vi "ChordsRecognition.vi"() -> ()   [LabVIEW 2021]
uses:
  <vilib>/Utility/NIReport.llb/Report Type.ctl
  <vilib>/numeric/Random Number (Range) I64.vi
  <vilib>/Analysis/baseanly.llb/Real A x B.vi
  <vilib>/numeric/sub_Random U32.vi
  <vilib>/Utility/file.llb/Read Delimited Spreadsheet (DBL).vi
  <vilib>/addons/_office/excel.llb/Excel Easy Table (str).vi
  <vilib>/Analysis/Matrix/Numeric/Conversions/Matrix To Array - RM.vi
  <vilib>/Utility/NIReport.llb/NI_report.lvclass
  <vilib>/Analysis/NI_AALBase.lvlib
  <vilib>/Analysis/Matrix/NI_Matrix.lvlib
  <vilib>/Utility/NIReport.llb/NI_ReportGenerationCore.lvlib
  <vilib>/Utility/NIReport.llb/Excel/NI_Excel.lvclass
  <vilib>/addons/_office/NI_ReportGenerationToolkit.lvlib
panel:
  out "n":i32
  in  "Save":bool
  in  "Array":bool[](array[boolean])
  in  "Saved":bool
  in  "index":i32
  out "Y_ideal":dbl[][][](array[numeric])
  out "Playing":string
  out "Keys":bool[][](array[boolean])
  out "la#":bool
  out "sol#":bool
  out "fa#":bool
  out "re#":bool
  out "do#":bool
  out "si":bool
  out "la":bool
  out "sol":bool
  out "fa":bool
  out "mi":bool
  out "re":bool
  out "do":bool
  out "Confidence":dbl
  out "min value":dbl
  out "max value":dbl
  in  "Random":bool
  in  "Output":i32=1
  in  "2th layer":i32=2
  in  "1th layer":i32=3
  in  "Predict":bool
  out "Error":dbl[](array[numeric])
  in  "W1":dbl[][](array[numeric])
  out "Y":dbl[][][](array[numeric])
  in  "Learn?":bool
  in  "Lr":dbl
  in  "stop":bool
  in  "Bias 2":dbl[][](array[numeric]) format="%#_13g"
  in  "Bias 3":dbl[][](array[numeric]) format="%#_13g"
  in  "Bias 1":dbl[][](array[numeric]) format="%#_13g"
  in  "W2":dbl[][](array[numeric])
  in  "W3":dbl[][](array[numeric])
  out "C":i16[][](array[numeric])
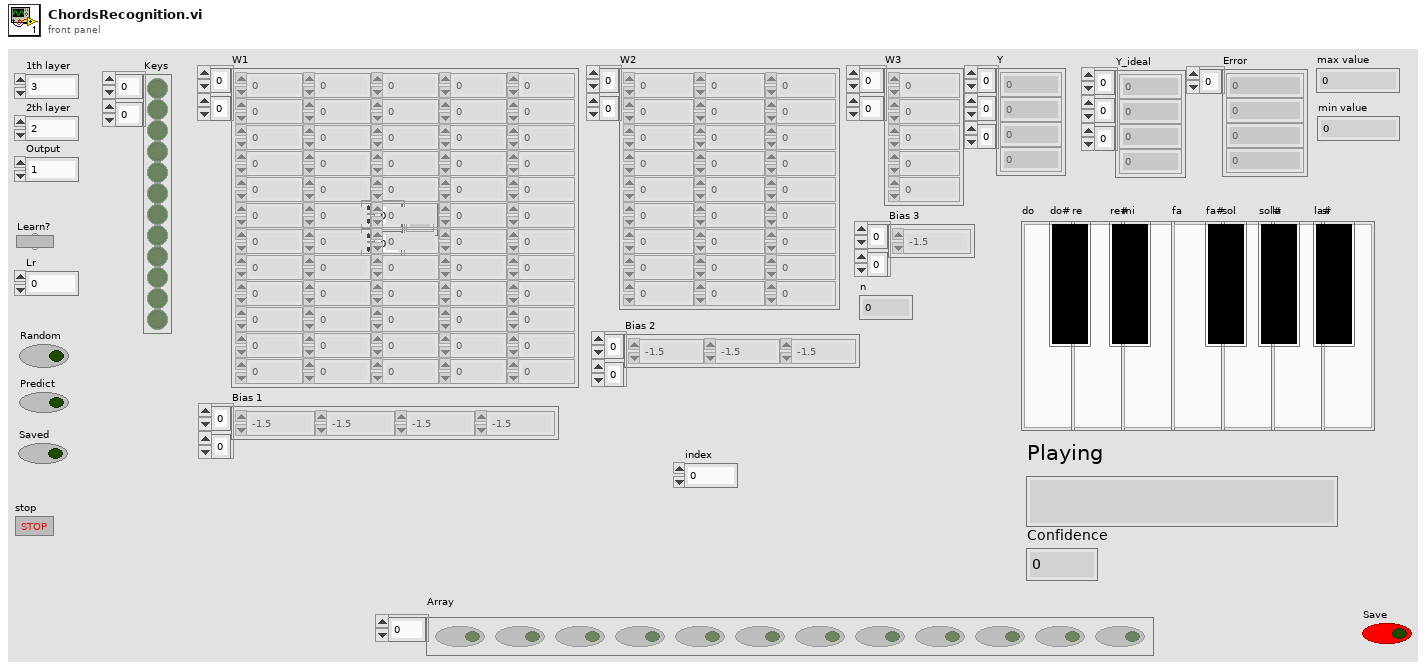
[diagram p1: front panel]
types:
  T1 = typedef "NI_ReportGenerationCore.lvlib/Report Type.ctl" = enum16{"HTML", "Word", "Excel"}
  T2 = typedef "NI_Matrix.lvlib/RealMatrix.ctl" = dbl[][]
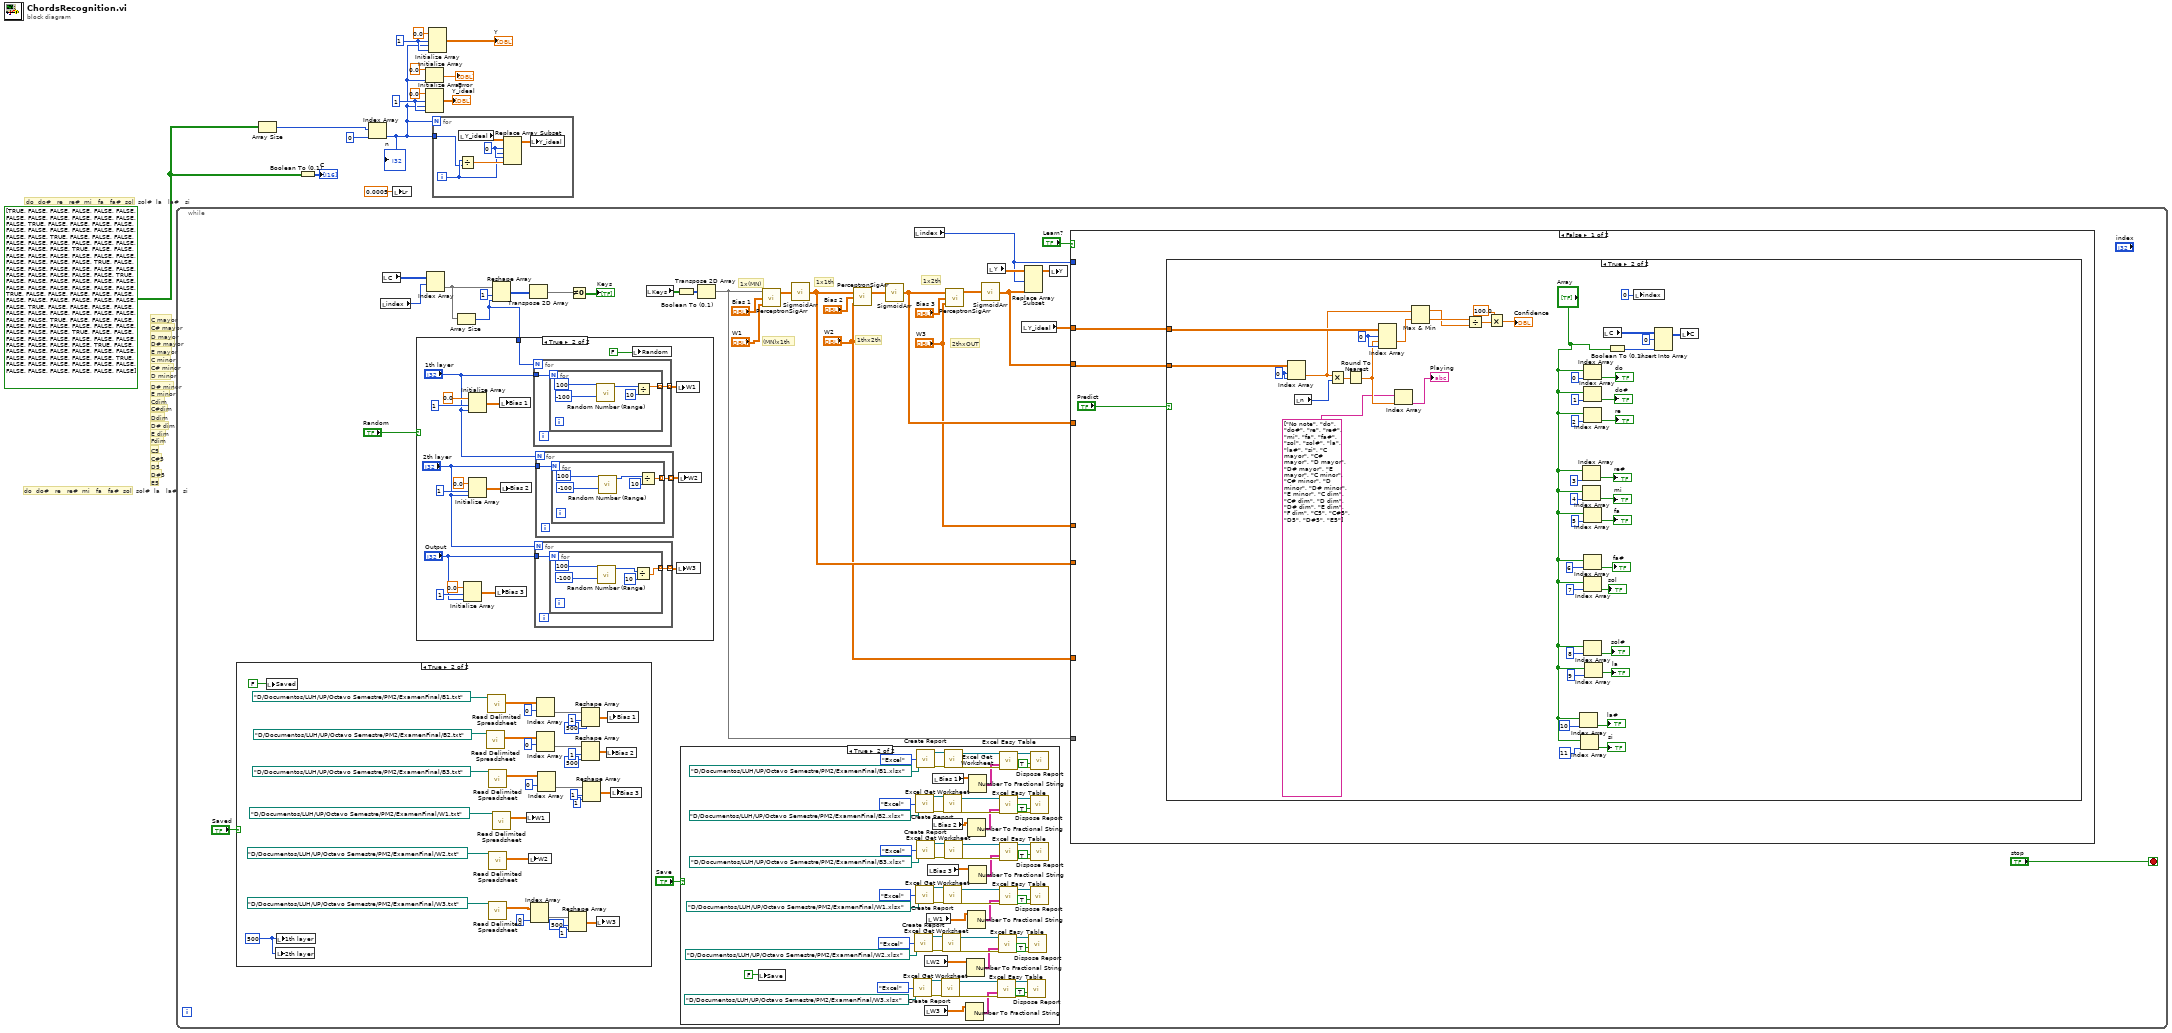
[diagram p0: block diagram]
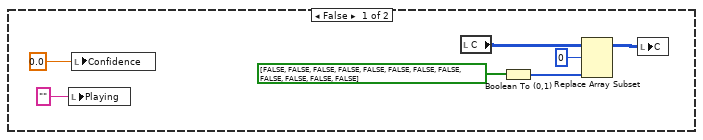
[diagram p5: hidden frame]
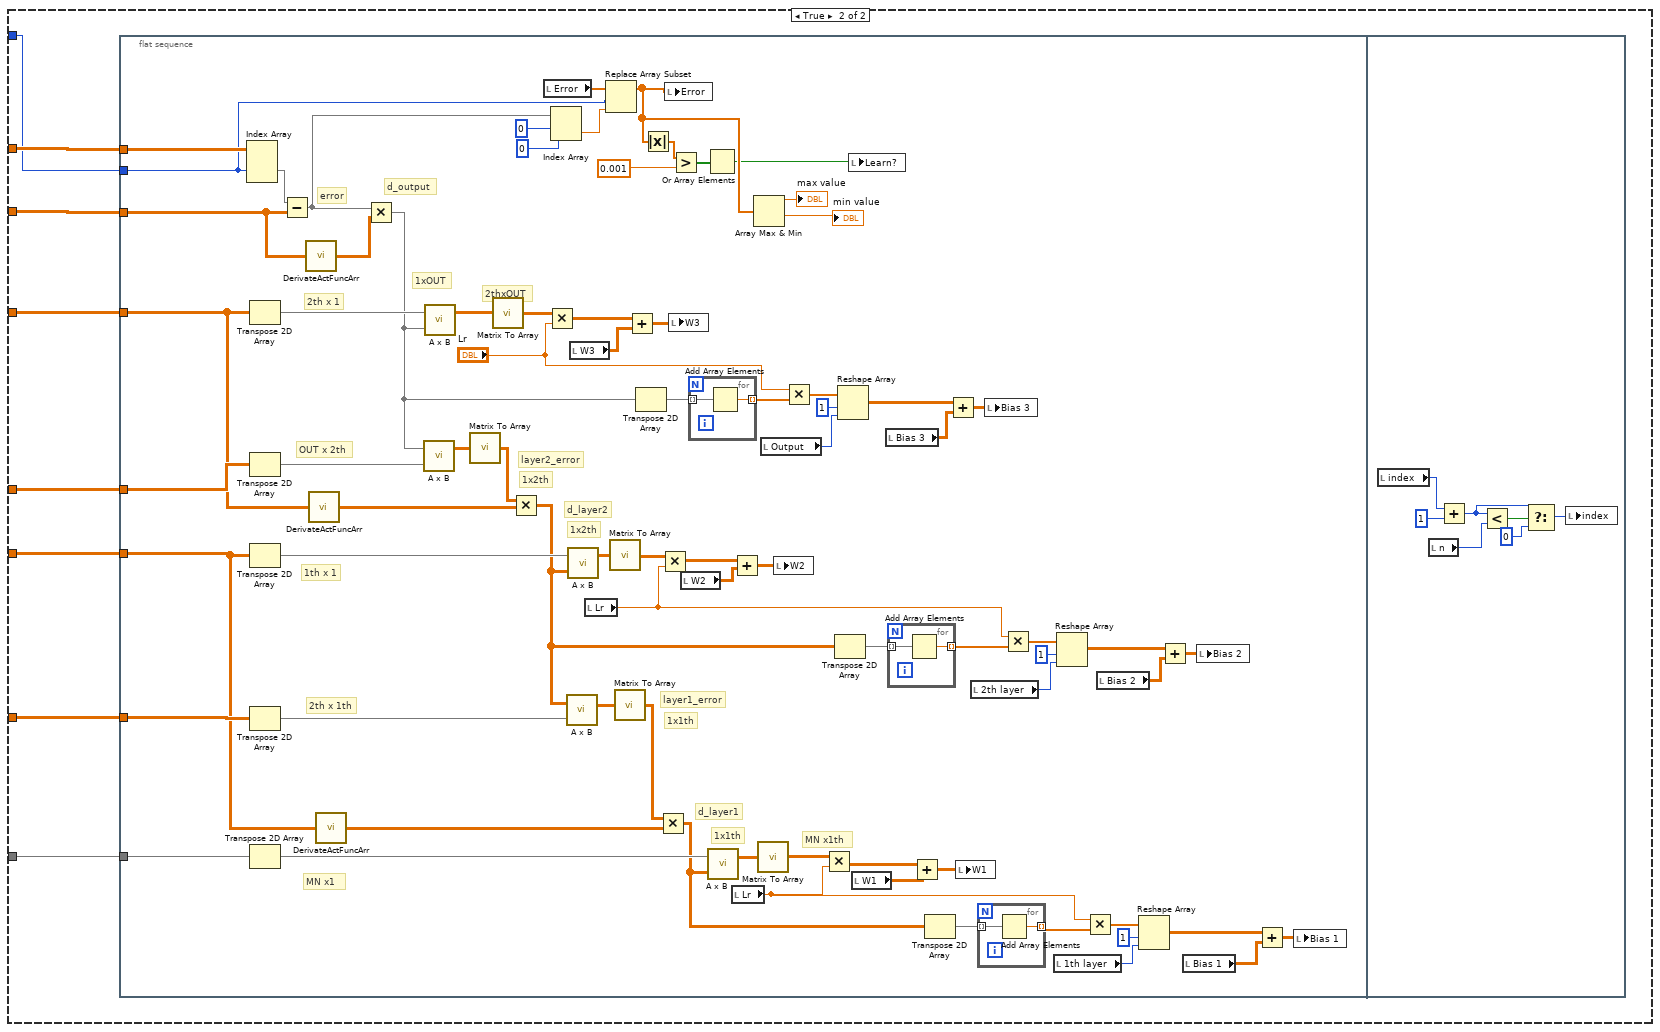
[diagram p6: hidden frame]
diagram:
  w1 = bool[][] [[TRUE, FALSE, FALSE, FALSE, FALSE, FALSE, FALSE, FALSE, FALSE, FALSE, FALSE, FALSE], [FALSE, TRUE, FALSE, FALSE, FALSE, FALSE, FALSE, FALSE, FALSE, FALSE, FALSE, FALSE], [FALSE, FALSE, TRUE, FALSE, FALSE, FALSE, FALSE, FALSE, FALSE, FALSE, FALSE, FALSE], [FALSE, FALSE, FALSE, TRUE, FALSE, FALSE, FALSE, FALSE, FALSE, FALSE, FALSE, FALSE], [FALSE, FALSE, FALSE, FALSE, TRUE, FALSE, FALSE, FALSE, FALSE, FALSE, FALSE, FALSE], [FALSE, FALSE, FALSE, FALSE, FALSE, TRUE, FALSE, FALSE, FALSE, FALSE, FALSE, FALSE], [FALSE, FALSE, FALSE, FALSE, FALSE, FALSE, TRUE, FALSE, FALSE, FALSE, FALSE, FALSE], [FALSE, FALSE, FALSE, FALSE, FALSE, FALSE, FALSE, TRUE, FALSE, FALSE, FALSE, FALSE], [FALSE, FALSE, FALSE, FALSE, FALSE, FALSE, FALSE, FALSE, TRUE, FALSE, FALSE, FALSE], [FALSE, FALSE, FALSE, FALSE, FALSE, FALSE, FALSE, FALSE, FALSE, TRUE, FALSE, FALSE], [FALSE, FALSE, FALSE, FALSE, FALSE, FALSE, FALSE, FALSE, FALSE, FALSE, TRUE, FALSE], [FALSE, FALSE, FALSE, FALSE, FALSE, FALSE, FALSE, FALSE, FALSE, FALSE, FALSE, TRUE], [FALSE, FALSE, FALSE, FALSE, FALSE, FALSE, FALSE, FALSE, FALSE, FALSE, FALSE, FALSE]]
  w7 = 1 ("dimension size")
  w13 = 1 ("dimension size")
  # "do  do#   re   re#  mi   fa   fa#  sol  sol#  la   la#   si"
  # "do  do#   re   re#  mi   fa   fa#  sol  sol#  la   la#   si"
  # "D# dim"
  # "D5"
  # "Ddim"
  # "C#5"
  # "C#dim"
  # "C5"
  # "Cdim"
  # "Fdim"
  # "E5"
  # "E dim"
  # "E minor"
  # "E mayor"
  # "D#5"
  # "D# minor"
  # "D# mayor"
  # "D minor"
  # "D mayor"
  # "C# minor"
  # "C# mayor"
  # "C minor"
  # "C mayor"
  n1 = while {
    stop <- "stop" stop-if-true
    # "2thxOUT"
    # "1x2th"
    # "1thx2th"
    # "1x1th"
    # "1x(MN)"
    # "(MN)x1th"
    n2 = case shown="True" "Saved" {
      frame False {
      }
      frame True {
        w140 = 500 ("1th layer")
        n3 = local write "Saved"(FALSE ("Boolean")) -> ()
        n4 = local write "2th layer"(w140) -> ()
        n5 = local write "1th layer"(w140) -> ()
        n6 = call-poly <vilib>:"Read Delimited Spreadsheet.vi"("file path (dialog if empty)"=path "D:/Documentos/LUH/UP/Octavo Semestre/PM2/ExamenFinal/B2.txt" ("template (empty)")) -> ("all rows"=w128:dbl[][])  [unwired: 9 in, 5 out]
        n7 = call-poly <vilib>:"Read Delimited Spreadsheet.vi"("file path (dialog if empty)"=path "D:/Documentos/LUH/UP/Octavo Semestre/PM2/ExamenFinal/B1.txt" ("template (empty)")) -> ("all rows"=w137:dbl[][])  [unwired: 9 in, 5 out]
        n8 = call-poly <vilib>:"Read Delimited Spreadsheet.vi"("file path (dialog if empty)"=path "D:/Documentos/LUH/UP/Octavo Semestre/PM2/ExamenFinal/B3.txt" ("template (empty)")) -> ("all rows"=w121:dbl[][])  [unwired: 9 in, 5 out]
        n9 = call-poly <vilib>:"Read Delimited Spreadsheet.vi"("file path (dialog if empty)"=path "D:/Documentos/LUH/UP/Octavo Semestre/PM2/ExamenFinal/W3.txt" ("template (empty)")) -> ("all rows"=w119:dbl[][])  [unwired: 9 in, 5 out]
        n10 = call-poly <vilib>:"Read Delimited Spreadsheet.vi"("file path (dialog if empty)"=path "D:/Documentos/LUH/UP/Octavo Semestre/PM2/ExamenFinal/W2.txt" ("template (empty)")) -> ("all rows"=w138:dbl[][])  [unwired: 9 in, 5 out]
        n11 = call-poly <vilib>:"Read Delimited Spreadsheet.vi"("file path (dialog if empty)"=path "D:/Documentos/LUH/UP/Octavo Semestre/PM2/ExamenFinal/W1.txt" ("template (empty)")) -> ("all rows"=w139:dbl[][])  [unwired: 9 in, 5 out]
        n12 = local write "W1"(w139) -> ()
        n13 = local write "W2"(w138) -> ()
        n14 = Index Array(array=w119, index (col)=0 ("index (row)")) -> (element=w116:dbl[])  [unwired: 1 in]
        n15 = Index Array(array=w137, index (row)=0) -> (element=w135:dbl[])  [unwired: 1 in]
        n16 = Index Array(array=w128, index (row)=0) -> (element=w130:dbl[])  [unwired: 1 in]
        n17 = Index Array(array=w121, index (row)=0) -> (element=w124:dbl[])  [unwired: 1 in]
        n18 = Reshape Array(w116, 500 ("dimension size"), 1 ("dimension size")) -> (w115:dbl[][])
        n19 = Reshape Array(w135, 1 ("dimension size"), 500 ("dimension size")) -> (w132:dbl[][])
        n20 = Reshape Array(w130, 1 ("dimension size"), 500 ("dimension size")) -> (w127:dbl[][])
        n21 = Reshape Array(w124, 1 ("dimension size"), 1 ("dimension size")) -> (w120:dbl[][])
        n22 = local write "W3"(w115) -> ()
        n23 = local write "Bias 2"(w127) -> ()
        n24 = local write "Bias 1"(w132) -> ()
        n25 = local write "Bias 3"(w120) -> ()
      }
    }
    n26 = local read "index"() -> (w17:i32)
    n27 = local read "C"() -> (w21:i16[][])
    n28 = Index Array(array=w21, index (row)=w17) -> (element=w16:i16[])  [unwired: 1 in]
    n29 = Array Size(array=w16) -> (size(s)=w15:i32)
    n30 = case shown="True" "Random" {
      tunnel: w15 -> [_ w163]
      frame False {
      }
      frame True {
        n31 = Initialize Array(0.0 ("element"), 1 ("dimension size"), "Output") -> (w148:dbl[][])
        n32 = Initialize Array(0.0 ("element"), 1 ("dimension size"), "1th layer") -> (w162:dbl[][])
        n33 = Initialize Array(0.0 ("element"), 1 ("dimension size"), "2th layer") -> (w157:dbl[][])
        n34 = local write "Bias 3"(w148) -> ()
        n35 = local write "Bias 1"(w162) -> ()
        n36 = local write "Bias 2"(w157) -> ()
        n37 = for {
          N: w163 -> [_]
          tunnel: "1th layer" -> [w180]
          tunnel: [w179] -> w159 mode=indexing
          n38 = for {
            N: w180 -> [_]
            tunnel: [w182] -> w179 mode=indexing
            n39 = call-poly <vilib>:"Random Number (Range).vi"("lower bound (-100)"=i64 -100, "upper bound (100)"=i64 100) -> ("number"=w183:i64)  [unwired: 9 in]
            n40 = Divide(x=w183, y=i64 10) -> (x/y=w182:dbl)
          }
        }
        n41 = for {
          N: "2th layer" -> [_]
          tunnel: "Output" -> [w166]
          tunnel: [w165] -> w152 mode=indexing
          n42 = for {
            N: w166 -> [_]
            tunnel: [w167] -> w165 mode=indexing
            n43 = call-poly <vilib>:"Random Number (Range).vi"("lower bound (-100)"=i64 -100, "upper bound (100)"=i64 100) -> ("number"=w168:i64)  [unwired: 9 in]
            n44 = Divide(x=w168, y=i64 10) -> (x/y=w167:dbl)
          }
        }
        n45 = for {
          N: "1th layer" -> [_]
          tunnel: "2th layer" -> [w173]
          tunnel: [w172] -> w153 mode=indexing
          n46 = for {
            N: w173 -> [_]
            tunnel: [w175] -> w172 mode=indexing
            n47 = call-poly <vilib>:"Random Number (Range).vi"("lower bound (-100)"=i64 -100, "upper bound (100)"=i64 100) -> ("number"=w174:i64)  [unwired: 9 in]
            n48 = Divide(x=w174, y=i64 10) -> (x/y=w175:dbl)
          }
        }
        n49 = local write "Random"(FALSE ("Init")) -> ()
        n50 = local write "W1"(w159) -> ()
        n51 = local write "W3"(w152) -> ()
        n52 = local write "W2"(w153) -> ()
      }
    }
    n53 = Reshape Array(w16, 1 ("dimension size"), w15) -> (w19:i16[][])
    n54 = Transpose 2D Array(2D array=w19) -> (transposed array=w18:i16[][])
    n55 = Not Equal To 0?(x=w18) -> (x != 0?=→"Keys":bool[][])
    n56 = local read "Keys"() -> (w29:bool[][])
    n57 = Boolean To (0,1)(Boolean=w29) -> (0, 1=w30:i16[][])
    n58 = case shown="True" "Save" {
      frame False {
      }
      frame True {
        n59 = local write "Save"(FALSE ("Save")) -> ()
        n60 = call <vilib>:"Create Report.vi"("report type"=Report_Type."Excel", "template (empty)"=path "D:/Documentos/LUH/UP/Octavo Semestre/PM2/ExamenFinal/W3.xlsx") -> ("report out"=w61:refnum<class "NI_report.lvclass">, "error out"=w60:errorcluster)  [unwired: 12 in]
        n61 = call <vilib>:"Create Report.vi"("report type"=Report_Type."Excel", "template (empty)"=path "D:/Documentos/LUH/UP/Octavo Semestre/PM2/ExamenFinal/W2.xlsx") -> ("report out"=w71:refnum<class "NI_report.lvclass">, "error out"=w70:errorcluster)  [unwired: 12 in]
        n62 = call <vilib>:"Create Report.vi"("report type"=Report_Type."Excel", "template (empty)"=path "D:/Documentos/LUH/UP/Octavo Semestre/PM2/ExamenFinal/B2.xlsx") -> ("report out"=w101:refnum<class "NI_report.lvclass">, "error out"=w100:errorcluster)  [unwired: 12 in]
        n63 = call <vilib>:"Create Report.vi"("report type"=Report_Type."Excel", "template (empty)"=path "D:/Documentos/LUH/UP/Octavo Semestre/PM2/ExamenFinal/W1.xlsx") -> ("report out"=w81:refnum<class "NI_report.lvclass">, "error out"=w80:errorcluster)  [unwired: 12 in]
        n64 = call <vilib>:"Create Report.vi"("report type"=Report_Type."Excel", "template (empty)"=path "D:/Documentos/LUH/UP/Octavo Semestre/PM2/ExamenFinal/B1.xlsx") -> ("report out"=w111:refnum<class "NI_report.lvclass">, "error out"=w110:errorcluster)  [unwired: 12 in]
        n65 = call <vilib>:"Create Report.vi"("report type"=Report_Type."Excel", "template (empty)"=path "D:/Documentos/LUH/UP/Octavo Semestre/PM2/ExamenFinal/B3.xlsx") -> ("report out"=w91:refnum<class "NI_report.lvclass">, "error out"=w90:errorcluster)  [unwired: 12 in]
        n66 = local read "W2"() -> (w49:dbl[][])
        n67 = local read "W3"() -> (w48:dbl[][])
        n68 = local read "W1"() -> (w50:dbl[][])
        n69 = local read "Bias 3"() -> (w51:dbl[][])
        n70 = local read "Bias 2"() -> (w52:dbl[][])
        n71 = local read "Bias 1"() -> (w53:dbl[][])
        n72 = call <vilib>:"Excel Get Worksheet.vi"("report in"=w61, "error in (no error)"=w60) -> ("report out"=w59:refnum<class "NI_report.lvclass">, "error out"=w58:errorcluster)  [unwired: 12 in]
        n73 = call <vilib>:"Excel Get Worksheet.vi"("report in"=w71, "error in (no error)"=w70) -> ("report out"=w69:refnum<class "NI_report.lvclass">, "error out"=w68:errorcluster)  [unwired: 12 in]
        n74 = call <vilib>:"Excel Get Worksheet.vi"("report in"=w101, "error in (no error)"=w100) -> ("report out"=w99:refnum<class "NI_report.lvclass">, "error out"=w98:errorcluster)  [unwired: 12 in]
        n75 = call <vilib>:"Excel Get Worksheet.vi"("report in"=w81, "error in (no error)"=w80) -> ("report out"=w79:refnum<class "NI_report.lvclass">, "error out"=w78:errorcluster)  [unwired: 12 in]
        n76 = call <vilib>:"Excel Get Worksheet.vi"("report in"=w111, "error in (no error)"=w110) -> ("report out"=w109:refnum<class "NI_report.lvclass">, "error out"=w108:errorcluster)  [unwired: 12 in]
        n77 = call <vilib>:"Excel Get Worksheet.vi"("report in"=w91, "error in (no error)"=w90) -> ("report out"=w89:refnum<class "NI_report.lvclass">, "error out"=w88:errorcluster)  [unwired: 12 in]
        n78 = Number To Fractional String(number=w48) -> (F-format string=w57:string[][])  [unwired: 3 in]
        n79 = Number To Fractional String(number=w49) -> (F-format string=w67:string[][])  [unwired: 3 in]
        n80 = Number To Fractional String(number=w52) -> (F-format string=w97:string[][])  [unwired: 3 in]
        n81 = Number To Fractional String(number=w50) -> (F-format string=w77:string[][])  [unwired: 3 in]
        n82 = Number To Fractional String(number=w53) -> (F-format string=w107:string[][])  [unwired: 3 in]
        n83 = Number To Fractional String(number=w51) -> (F-format string=w87:string[][])  [unwired: 3 in]
        n84 = call-poly <vilib>:"Excel Easy Table.vi"("report in"=w59, "text data"=w57, "error in (no error)"=w58) -> ("report out"=w56:refnum<class "NI_report.lvclass">, "error out"=w55:errorcluster)  [unwired: 8 in, 3 out]
        n85 = call-poly <vilib>:"Excel Easy Table.vi"("report in"=w69, "text data"=w67, "error in (no error)"=w68) -> ("report out"=w66:refnum<class "NI_report.lvclass">, "error out"=w65:errorcluster)  [unwired: 8 in, 3 out]
        n86 = call-poly <vilib>:"Excel Easy Table.vi"("report in"=w99, "text data"=w97, "error in (no error)"=w98) -> ("report out"=w96:refnum<class "NI_report.lvclass">, "error out"=w95:errorcluster)  [unwired: 8 in, 3 out]
        n87 = call-poly <vilib>:"Excel Easy Table.vi"("report in"=w79, "text data"=w77, "error in (no error)"=w78) -> ("report out"=w76:refnum<class "NI_report.lvclass">, "error out"=w75:errorcluster)  [unwired: 8 in, 3 out]
        n88 = call-poly <vilib>:"Excel Easy Table.vi"("report in"=w109, "text data"=w107, "error in (no error)"=w108) -> ("report out"=w106:refnum<class "NI_report.lvclass">, "error out"=w105:errorcluster)  [unwired: 8 in, 3 out]
        n89 = call-poly <vilib>:"Excel Easy Table.vi"("report in"=w89, "text data"=w87, "error in (no error)"=w88) -> ("report out"=w86:refnum<class "NI_report.lvclass">, "error out"=w85:errorcluster)  [unwired: 8 in, 3 out]
        n90 = call-dynamic "Dispose Report.vi"("report in"=w56, "save changes? (F)"=TRUE, "error in (no error)"=w55) -> ()  [unwired: 12 in, 1 out]
        n91 = call-dynamic "Dispose Report.vi"("report in"=w66, "save changes? (F)"=TRUE, "error in (no error)"=w65) -> ()  [unwired: 12 in, 1 out]
        n92 = call-dynamic "Dispose Report.vi"("report in"=w96, "save changes? (F)"=TRUE, "error in (no error)"=w95) -> ()  [unwired: 12 in, 1 out]
        n93 = call-dynamic "Dispose Report.vi"("report in"=w76, "save changes? (F)"=TRUE, "error in (no error)"=w75) -> ()  [unwired: 12 in, 1 out]
        n94 = call-dynamic "Dispose Report.vi"("report in"=w106, "save changes? (F)"=TRUE, "error in (no error)"=w105) -> ()  [unwired: 12 in, 1 out]
        n95 = call-dynamic "Dispose Report.vi"("report in"=w86, "save changes? (F)"=TRUE, "error in (no error)"=w85) -> ()  [unwired: 12 in, 1 out]
      }
    }
    n96 = Transpose 2D Array(2D array=w30) -> (transposed array=w28:i16[][])
    n97 = call "PerceptronSigArr.vi"("Wa"="W1", "Bias"="Bias 1", "Xa"=w28) -> ("Y"=w41:dbl[][])
    n98 = call "SigmoidArr.vi"("x"=w41) -> ("Sigmoid"=w38:dbl[][])
    n99 = call "PerceptronSigArr.vi"("Wa"="W2", "Bias"="Bias 2", "Xa"=w38) -> ("Y"=w44:dbl[][])
    n100 = call "SigmoidArr.vi"("x"=w44) -> ("Sigmoid"=w36:dbl[][])
    n101 = local read "index"() -> (w26:i32)
    n102 = call "PerceptronSigArr.vi"("Wa"="W3", "Bias"="Bias 3", "Xa"=w36) -> ("Y"=w42:dbl[][])
    n103 = call "SigmoidArr.vi"("x"=w42) -> ("Sigmoid"=w25:dbl[][])
    n104 = local read "Y"() -> (w27:dbl[][][])
    n105 = local read "Y_ideal"() -> (w23:dbl[][][])
    n106 = Replace Array Subset(array=w27, new element=w25, index (dim 1)=w26) -> (w24:dbl[][][])  [unwired: 2 in]
    n107 = local write "Y"(w24) -> ()
    n108 = case shown="False" "Learn?" {
      tunnel: w25 -> [w187 w248]
      tunnel: w23 -> [w186 w249]
      tunnel: w36 -> [_ w246]
      tunnel: "W3" -> [_ w247]
      tunnel: w38 -> [_ w244]
      tunnel: "W2" -> [_ w245]
      tunnel: w28 -> [_ w243]
      tunnel: w26 -> [_ w242]
      frame False {
        n109 = case shown="True" "Predict" {
          tunnel: w187 -> [_ w240]
          tunnel: w186 -> [_ w239]
          frame False {
            n110 = local write "Playing"("" ("Playing")) -> ()
            n111 = local write "Confidence"(0.0 ("Pattern")) -> ()
            n112 = local read "C"() -> (w191:i16[][])
            n113 = Boolean To (0,1)(Boolean=bool[] [FALSE, FALSE, FALSE, FALSE, FALSE, FALSE, FALSE, FALSE, FALSE, FALSE, FALSE, FALSE]) -> (0, 1=w193:i16[])
            n114 = Replace Array Subset(array=w191, new element=w193, index (row)=0) -> (w189:i16[][])  [unwired: 1 in]
            n115 = local write "C"(w189) -> ()
          }
          frame True {
            w238 = 0 ("disabled index (page)")
            w241 = 0 ("index (row)")
            n116 = Index Array(array=w240, index (row)=w241, index (col)=w241) -> (element=w230:dbl)
            n117 = local read "n"() -> (w196:i32)
            n118 = Multiply(x=w230, y=w196) -> (x*y=w234:dbl)
            n119 = Round To Nearest(number=w234) -> (nearest integer value=w229:dbl)
            n120 = Index Array(array=w239, index (dim 0)=w238, index (dim 1)=w229, index (dim 2)=w238) -> (element=w231:dbl)
            n121 = Index Array(array=string[] ["No note", "do", "do#", "re", "re#", "mi", "fa", "fa#", "sol", "sol#", "la", "la#", "si", "C mayor", "C# mayor", "D mayor", "D# mayor", "E mayor", "C minor", "C# minor", "D minor", "D# minor", "E minor", "C dim", "C# dim", "D dim", "D# dim", "E dim", "F dim", "C5", "C#5", "D5", "D#5", "E5"], index=w229) -> (element=→"Playing":string)
            n122 = Max & Min(x=w230, y=w231) -> (max(x,y)=w232:dbl, min(x,y)=w233:dbl)
            n123 = Divide(x=w233, y=w232) -> (x/y=w237:dbl)
            n124 = Multiply(x=100.0, y=w237) -> (x*y=→"Confidence":dbl)
            n125 = Index Array(array="Array", index=10) -> (element=→"la#":bool)
            n126 = Index Array(array="Array", index=11) -> (element=→"si":bool)
            n127 = Index Array(array="Array", index=3) -> (element=→"re#":bool)
            n128 = Index Array(array="Array", index=4) -> (element=→"mi":bool)
            n129 = Index Array(array="Array", index=0) -> (element=→"do":bool)
            n130 = Index Array(array="Array", index=2) -> (element=→"re":bool)
            n131 = Index Array(array="Array", index=5) -> (element=→"fa":bool)
            n132 = Index Array(array="Array", index=6) -> (element=→"fa#":bool)
            n133 = Index Array(array="Array", index=1) -> (element=→"do#":bool)
            n134 = Index Array(array="Array", index=7) -> (element=→"sol":bool)
            n135 = Index Array(array="Array", index=8) -> (element=→"sol#":bool)
            n136 = Index Array(array="Array", index=9) -> (element=→"la":bool)
            n137 = local read "C"() -> (w202:i16[][])
            n138 = Boolean To (0,1)(Boolean="Array") -> (0, 1=w201:i16[])
            n139 = local write "index"(0 ("index")) -> ()
            n140 = Insert Into Array(array=w202, index (row)=0, new element=w201) -> (w199:i16[][])  [unwired: 1 in]
            n141 = local write "C"(w199) -> ()
          }
        }
      }
      frame True {
        n142 = flat-sequence {
          tunnel: w249 -> [w327]
          tunnel: w248 -> [w326]
          tunnel: w247 -> [w325]
          tunnel: w246 -> [w324]
          tunnel: w245 -> [w323]
          tunnel: w244 -> [w322]
          tunnel: w243 -> [w321]
          tunnel: w242 -> [w252]
          frame #0 {
            # "MN x1th"
            # "MN x1"
            # "1x1th"
            # "d_layer1"
            # "1x1th"
            # "layer1_error"
            # "2th x 1th"
            # "1th x 1"
            # "1x2th"
            # "OUT x 2th"
            # "d_layer2"
            # "1x2th"
            # "layer2_error"
            # "2thxOUT"
            # "1xOUT"
            # "2th x 1"
            # "d_output"
            # "error"
            n143 = Index Array(array=w327, index (dim 1)=w252) -> (element=w264:dbl[][])  [unwired: 2 in]
            n144 = Transpose 2D Array(2D array=w324) -> (transposed array=w307:dbl[][])
            n145 = Transpose 2D Array(2D array=w325) -> (transposed array=w297:dbl[][])
            n146 = Transpose 2D Array(2D array=w322) -> (transposed array=w293:dbl[][])
            n147 = Transpose 2D Array(2D array=w323) -> (transposed array=w282:dbl[][])
            n148 = Transpose 2D Array(2D array=w321) -> (transposed array=w278:i16[][])
            n149 = Subtract(x=w264, y=w326) -> (x-y=w259:dbl[][])
            n150 = call "DerivateActFuncArr.vi"("Input"=w326) -> ("Output"=w308:dbl[][])
            n151 = call "DerivateActFuncArr.vi"("Input"=w324) -> ("Output"=w296:dbl[][])
            n152 = call "DerivateActFuncArr.vi"("Input"=w322) -> ("Output"=w279:dbl[][])
            n153 = Multiply(x=w259, y=w308) -> (x*y=w266:dbl[][])
            n154 = call-poly <vilib>:"A x B.vi"("B"=w297, "A"=w266) -> ("A x B"=w295:T2)  [unwired: 1 out]
            n155 = call-poly <vilib>:"A x B.vi"("B"=w266, "A"=w307) -> ("A x B"=w306:T2)  [unwired: 1 out]
            n156 = call-poly <vilib>:"Matrix To Array.vi"("Real Matrix"=w295) -> ("Real 2D Array"=w294:dbl[][])
            n157 = call-poly <vilib>:"Matrix To Array.vi"("Real Matrix"=w306) -> ("Real 2D Array"=w305:dbl[][])
            n158 = Multiply ("Multiply.vi")(x=w294, y=w296) -> (x*y=w283:dbl[][])
            n159 = local read "Error"() -> (w265:dbl[])
            n160 = Multiply ("Multiply.vi")(x=w305, y="Lr") -> (x*y=w304:dbl[][])
            n161 = Index Array(array=w259, index (row)=0 ("index"), index (col)=0 ("disabled index (col)")) -> (element=w260:dbl)
            n162 = call-poly <vilib>:"A x B.vi"("B"=w282, "A"=w283) -> ("A x B"=w281:T2)  [unwired: 1 out]
            n163 = call-poly <vilib>:"A x B.vi"("B"=w283, "A"=w293) -> ("A x B"=w292:T2)  [unwired: 1 out]
            n164 = local read "W3"() -> (w318:dbl[][])
            n165 = local read "Lr"() -> (w262:dbl)
            n166 = Replace Array Subset(array=w265, new element=w260, index=w252) -> (w251:dbl[])
            n167 = call-poly <vilib>:"Matrix To Array.vi"("Real Matrix"=w292) -> ("Real 2D Array"=w291:dbl[][])
            n168 = call-poly <vilib>:"Matrix To Array.vi"("Real Matrix"=w281) -> ("Real 2D Array"=w280:dbl[][])
            n169 = Add ("Add.vi")(x=w304, y=w318) -> (x+y=w317:dbl[][])
            n170 = Transpose 2D Array(2D array=w266) -> (transposed array=w303:dbl[][])
            n171 = Absolute Value(x=w251) -> (abs(x)=w255:dbl[])
            n172 = Multiply ("Multiply.vi")(x=w280, y=w279) -> (x*y=w273:dbl[][])
            n173 = Multiply ("Multiply.vi")(x=w291, y=w262) -> (x*y=w290:dbl[][])
            n174 = local write "Error"(w251) -> ()
            n175 = local write "W3"(w317) -> ()
            n176 = Greater?(x=w255, y=0.001 ("x")) -> (0:w254:bool[])
            n177 = local read "W2"() -> (w313:dbl[][])
            n178 = for {
              tunnel: w303 -> [w333] mode=indexing
              tunnel: [w332] -> w302 mode=indexing
              n179 = Add Array Elements(numeric array=w333) -> (sum=w332:dbl)
            }
            n180 = Or Array Elements(Boolean array=w254) -> (logical OR=w250:bool)
            n181 = call-poly <vilib>:"A x B.vi"("B"=w273, "A"=w278) -> ("A x B"=w277:T2)  [unwired: 1 out]
            n182 = Add ("Add.vi")(x=w290, y=w313) -> (x+y=w314:dbl[][])
            n183 = local read "Lr"() -> (w269:dbl)
            n184 = Array Max & Min(array=w251) -> (max value=→"max value":dbl, min value=→"min value":dbl)  [unwired: 2 out]
            n185 = call-poly <vilib>:"Matrix To Array.vi"("Real Matrix"=w277) -> ("Real 2D Array"=w276:dbl[][])
            n186 = local read "Output"() -> (w299:i32)
            n187 = local write "W2"(w314) -> ()
            n188 = Multiply ("Multiply.vi")(x="Lr", y=w302) -> (x*y=w301:dbl[])
            n189 = Multiply ("Multiply.vi")(x=w276, y=w269) -> (x*y=w275:dbl[][])
            n190 = Transpose 2D Array(2D array=w283) -> (transposed array=w289:dbl[][])
            n191 = Reshape Array(w301, 1 ("dimension size"), w299) -> (w298:dbl[][])
            n192 = local write "Learn?"(w250) -> ()
            n193 = local read "W1"() -> (w320:dbl[][])
            n194 = local read "Bias 3"() -> (w316:dbl[][])
            n195 = for {
              tunnel: w289 -> [w331] mode=indexing
              tunnel: [w330] -> w285 mode=indexing
              n196 = Add Array Elements(numeric array=w331) -> (sum=w330:dbl)
            }
            n197 = Add(x=w275, y=w320) -> (x+y=w319:dbl[][])
            n198 = Transpose 2D Array(2D array=w273) -> (transposed array=w274:dbl[][])
            n199 = Add(x=w298, y=w316) -> (x+y=w315:dbl[][])
            n200 = local write "W1"(w319) -> ()
            n201 = local read "2th layer"() -> (w286:i32)
            n202 = for {
              tunnel: w274 -> [w329] mode=indexing
              tunnel: [w328] -> w270 mode=indexing
              n203 = Add Array Elements(numeric array=w329) -> (sum=w328:dbl)
            }
            n204 = local write "Bias 3"(w315) -> ()
            n205 = Multiply ("Multiply.vi")(x=w262, y=w285) -> (x*y=w288:dbl[])
            n206 = local read "1th layer"() -> (w268:i32)
            n207 = Reshape Array(w288, 1 ("dimension size"), w286) -> (w284:dbl[][])
            n208 = Multiply ("Multiply.vi")(x=w269, y=w270) -> (x*y=w272:dbl[])
            n209 = local read "Bias 2"() -> (w312:dbl[][])
            n210 = Reshape Array(w272, 1 ("dimension size"), w268) -> (w267:dbl[][])
            n211 = Add(x=w284, y=w312) -> (x+y=w311:dbl[][])
            n212 = local read "Bias 1"() -> (w310:dbl[][])
            n213 = local write "Bias 2"(w311) -> ()
            n214 = Add(x=w267, y=w310) -> (x+y=w309:dbl[][])
            n215 = local write "Bias 1"(w309) -> ()
          }
          frame #1 {
            n216 = local read "index"() -> (w340:i32)
            n217 = local read "n"() -> (w334:i32)
            n218 = Add(x=w340, y=1) -> (x+y=w339:i32)
            n219 = Less?(x=w339, y=w334) -> (x < y?=w338:bool)
            n220 = Select(t=w339, s=w338, f=0) -> (s? t:f=w335:i32)
            n221 = local write "index"(w335) -> ()
          }
        }
      }
    }
  }
  n222 = Array Size(array=w1) -> (size(s)=w10:i32[])
  n223 = Boolean To (0,1)(Boolean=w1) -> (0, 1=→"C":i16[][])
  n224 = Index Array(array=w10, index=0) -> (element=w2:i32)
  "n" <- w2
  n225 = local write "Lr"(0.0005 ("Lr")) -> ()
  n226 = Initialize Array(0.0 ("element"), w2) -> (→"Error":dbl[])
  n227 = Initialize Array(0.0 ("element"), w13, w2, w13) -> (→"Y_ideal":dbl[][][])
  n228 = Initialize Array(0.0 ("element"), w7, w2, w7) -> (→"Y":dbl[][][])
  n229 = for {
    N: w2 -> [_]
    tunnel: w2 -> [w341]
    i -> [w342]
    w344 = 0 ("index (page)")
    n230 = local read "Y_ideal"() -> (w345:dbl[][][])
    n231 = Divide(x=w342, y=w341) -> (x/y=w343:dbl)
    n232 = Replace Array Subset(array=w345, new element=w343, index (dim 0)=w344, index (dim 1)=w342, index (dim 2)=w344) -> (w346:dbl[][][])
    n233 = local write "Y_ideal"(w346) -> ()
  }
